vi "Get VI Name for API Call.vi"(8 "error in":errorcluster, 9 "API Call":T9, 11 "Hardware Configuration in":T1) -> (0 "error out":errorcluster, 3 "Hardware Configuration out":T1, 5 "VI Name":string)   [LabVIEW 2021, in "Acquisition.lvlib"]
doc: "Return the name of the VI for the matching 'API' and 'API Call'."
uses:
  Acquisition.lvlib
  API Call.ctl
  Hardware Configuration.ctl
  Channel Settings.ctl
  IO Device.ctl
  Sensor Type.ctl
  Interval Timer/Repeat Interval.ctl
  Interval Timer/Interval Length.ctl
  Interval Timer/Interval Token.ctl
  IO API.ctl
  Interval Timer/Interval Timer.lvlib
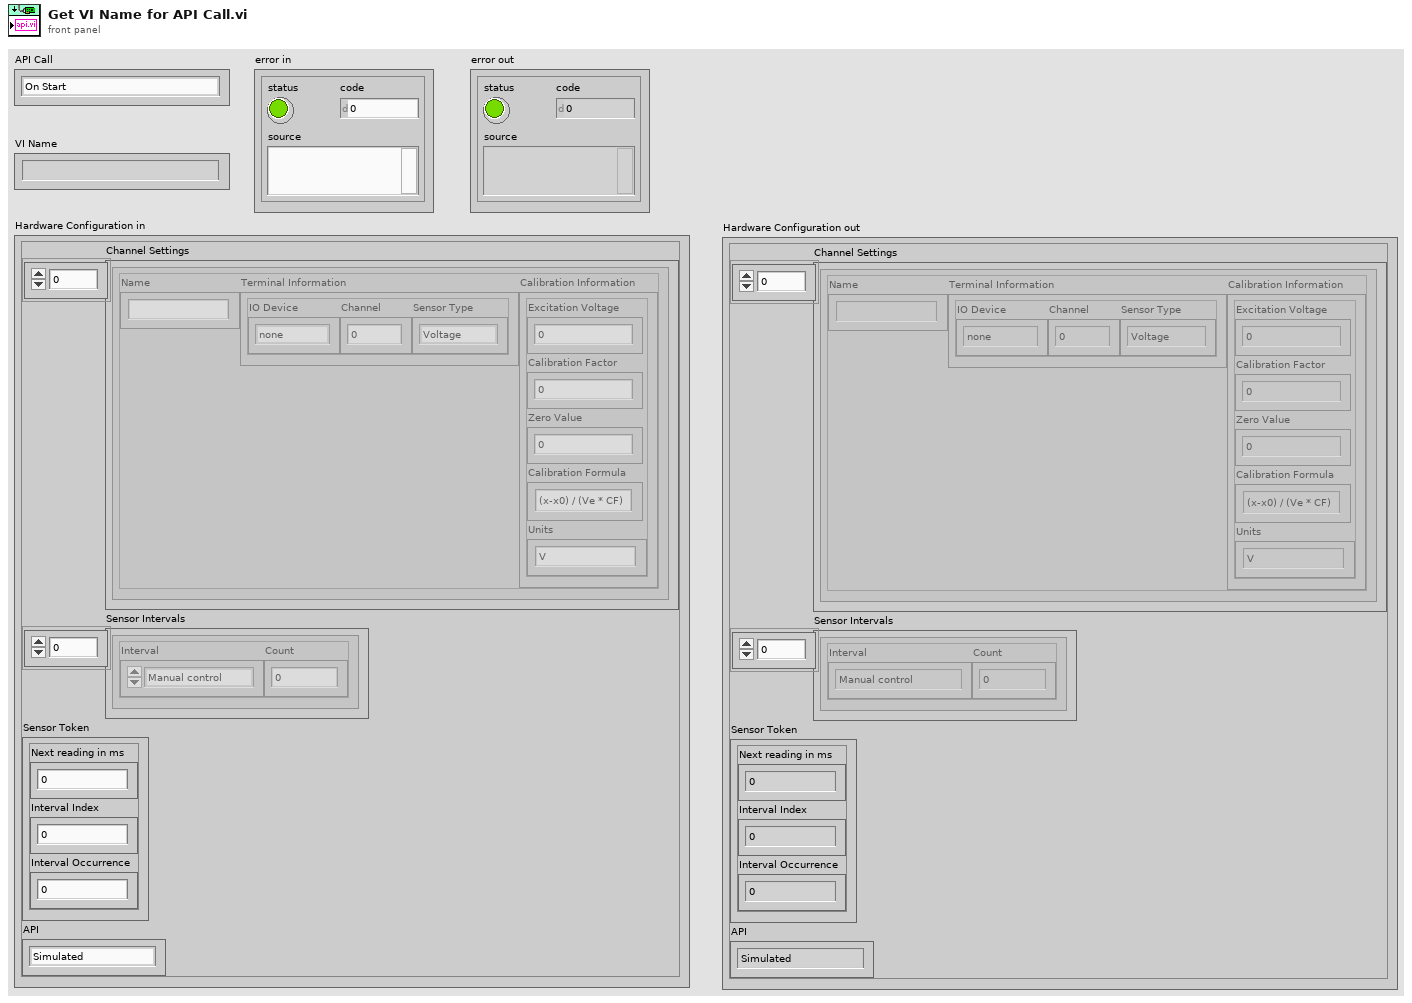
[diagram p1: front panel]
types:
  T1 = typedef "Acquisition.lvlib/Hardware Configuration.ctl" = cluster{"Channel Settings":T2[], "Sensor Intervals":T5[], "Sensor Token":T7, "API":T8}
  T2 = typedef "Acquisition.lvlib/Channel Settings.ctl" = cluster{"Name":string, "Terminal Information":cluster{"IO Device":T3, "Channel":i32, "Sensor Type":T4}, "Calibration Information":cluster{"Excitation Voltage":dbl, "Calibration Factor":dbl, "Zero Value":dbl, "Calibration Formula":string, "Units":string}}
  T3 = typedef "Acquisition.lvlib/IO Device.ctl" = enum16{"none", "9219", "9401"}
  T4 = typedef "Acquisition.lvlib/Sensor Type.ctl" = enum16{"Voltage", "Load", "Pressure", "Encoder"}
  T5 = typedef "Interval Timer.lvlib/Repeat Interval.ctl" = cluster{"Interval":T6, "Count":i32}
  T6 = typedef "Interval Timer.lvlib/Interval Length.ctl" = enum16{"Manual control", "1 second", "10 seconds", "30 seconds", "60 seconds", "600 seconds", "1200 seconds", "3600 seconds"}
  T7 = typedef "Interval Timer.lvlib/Interval Token.ctl" = cluster{"Next reading in ms":u32, "Interval Index":i32, "Interval Occurrence":i32}
  T8 = typedef "Acquisition.lvlib/IO API.ctl" = enum16{"Simulated", "DAQmx"}
  T9 = typedef "Acquisition.lvlib/API Call.ctl" = enum16{"On Start", "Acquire", "On Stop", "Preview"}
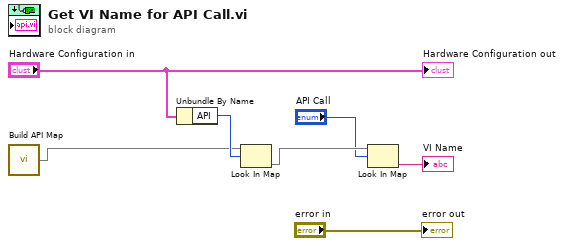
[diagram p0: block diagram]
diagram:
  n1 = call "Build API Map.vi"() -> ("API map"=w1:map{T8, map{T9, string}})
  n2 = Unbundle By Name("Hardware Configuration in") -> ("API"=w3:T8)
  n3 = Look In Map(map=w1, key=w3) -> (value=w7:map{T9, string})  [unwired: 1 in, 1 out]
  n4 = Look In Map(map=w7, key="API Call") -> (value=→"VI Name":string)  [unwired: 1 in, 1 out]
  "error out" <- "error in"
  "Hardware Configuration out" <- "Hardware Configuration in"
